vi "TFT SCan.vi"(4 "Scan Data":string, 5 "FTT":string) -> (1 "OutputData":string)   [LabVIEW 2015]
panel:
  # "6003103A4P973090Y07419-08-11TM035HFHP30-01"
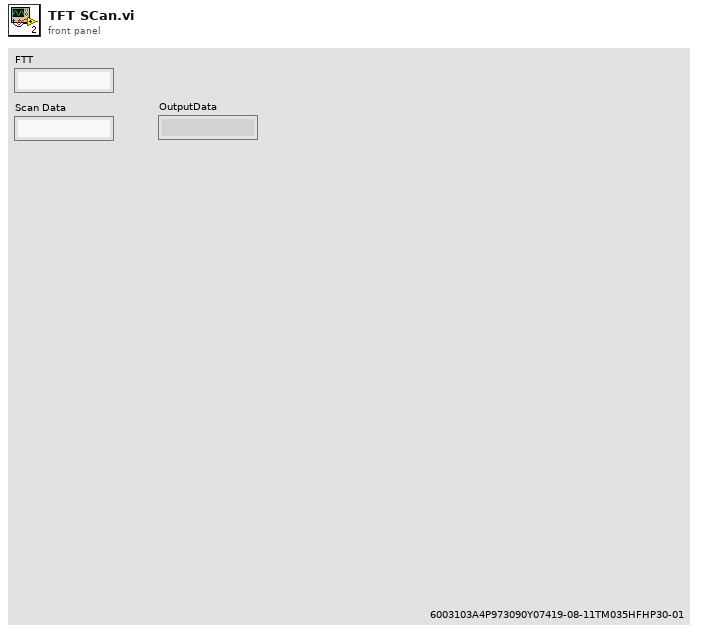
[diagram p1: front panel]
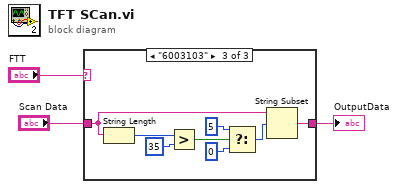
[diagram p0: block diagram]
diagram:
  n1 = case shown="\"6003103\"" "FTT" {
    tunnel: [w4 w5 w8] -> w2
    tunnel: "Scan Data" -> [w4 w5 w7]
    frame "False", Default {
    }
    frame "6530300" {
    }
    frame "6003103" {
      n2 = String Length(string=w7) -> (length=w6:i32)
      n3 = Greater?(x=w6, y=35) -> (0:w12:bool)
      n4 = Select(t=5 ("y"), s=w12, f=0) -> (s? t:f=w9:i32)
      n5 = String Subset(string=w7, offset (0)=w9) -> (substring=w8:string)  [unwired: 1 in]
    }
  }
  "OutputData" <- w2
